vi "getDefaultValue.vi"(8 "error in (no error)":errorcluster, 11 "IProperty in":refnum<class "IProperty.lvclass">) -> (0 "error out":errorcluster, 2 "Default Value out":refnum<class "IBaseObject.lvclass">, 3 "IProperty out":refnum<class "IProperty.lvclass">)   [LabVIEW 2022 SP3, in "openDAQ.lvlib" / "IBaseObject.lvlib" / "IProperty.lvlib" / "IProperty.lvclass"]
uses:
  <instrlib>/openDAQ/Public/Classes/IProperty/IProperty.lvclass
  <instrlib>/openDAQ/Public/Classes/IProperty/IProperty.lvclass/IProperty.ctl
  <instrlib>/openDAQ/Public/Classes/IBaseObject/IBaseObject.lvclass
  <instrlib>/openDAQ/Binaries/Windows/x86/copendaq32.dll
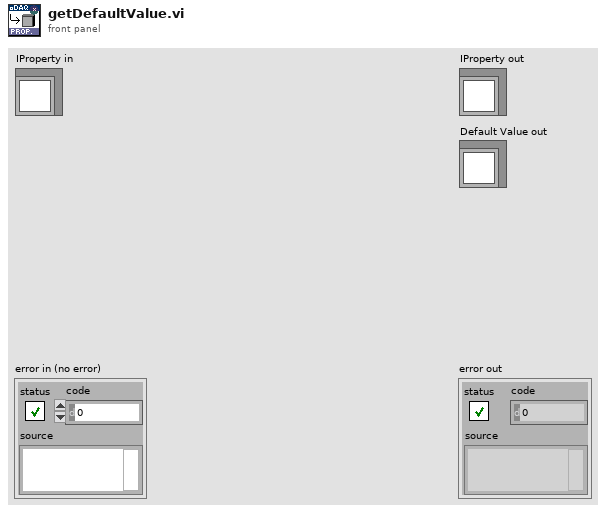
[diagram p1: front panel]
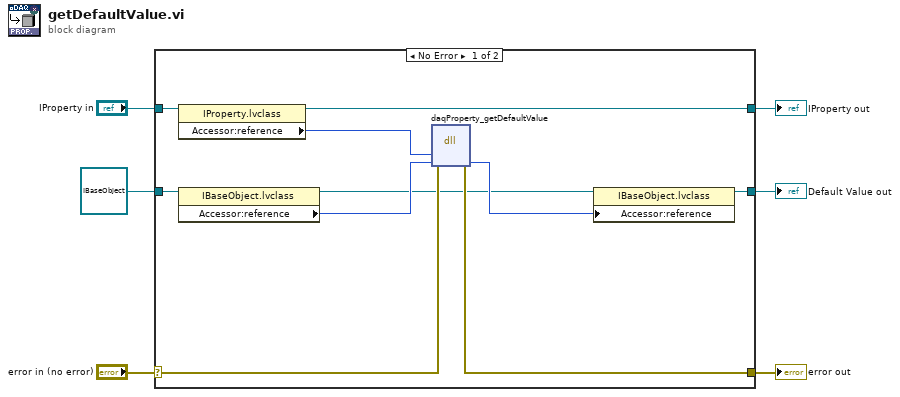
[diagram p0: block diagram]
diagram:
  n1 = case shown="No Error" "error in (no error)" {
    selector: "error in (no error)" -> [w14 w19]
    tunnel: [w13 w19] -> w5
    tunnel: [w9 w18] -> w3
    tunnel: "IProperty in" -> [w15 w18]
    tunnel: refnum<class "IBaseObject.lvclass"> refnum ("openDAQ.lvlib:IBaseObject.lvlib:IBaseObject.lvclass") -> [w12 w17]
    tunnel: [w7 w17] -> w1
    frame No Error {
      n2 = property class="IProperty.lvclass"(reference=w15) -> (reference out=w9:refnum<class "IProperty.lvclass">, "Accessor:reference"=w11:i64)  [unwired: 1 in, 1 out]
      n3 = property class="IBaseObject.lvclass"(reference=w12) -> (reference out=w8:refnum<class "IBaseObject.lvclass">, "Accessor:reference"=w10:i64)  [unwired: 1 in, 1 out]
      n4 = dll-call lib="C:/Program Files (x86)/National Instruments/LabVIEW 2022/instr.lib/openDAQ/Binaries/Windows/x86/copendaq*.*" fn="daqProperty_getDefaultValue"(error in=w14, "property"=w11, "defaultValue"=w10) -> (error out=w13:errorcluster, "defaultValue"=w16:i64)  [unwired: 4 in, 1 out]
      n5 = property class="IBaseObject.lvclass"(reference=w8, "Accessor:reference"=w16) -> (reference out=w7:refnum<class "IBaseObject.lvclass">)  [unwired: 1 in, 1 out]
    }
    frame Error {
    }
  }
  "error out" <- w5
  "IProperty out" <- w3
  "Default Value out" <- w1
